vi "Media Player Example.vi"() -> ()   [LabVIEW 2017]
uses:
  Audio Player/AudioPlayer.lvclass
panel:
  in  "fileName":string[](array[string])=["beyond the horizon.mp3", "alone.mp4", "far far away.vlc", "mind me.avi"]
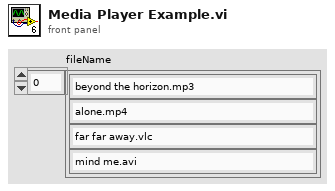
[diagram p1: front panel]
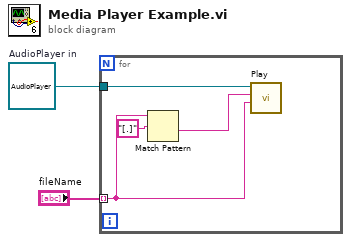
[diagram p0: block diagram]
diagram:
  w1 = refnum<class "AudioPlayer.lvclass"> refnum  # AudioPlayer in
  n1 = for {
    tunnel: "fileName" -> [w3] mode=indexing
    tunnel: w1 -> [w6]
    n2 = Match Pattern(string=w3, regular expression="[.]") -> (after substring=w4:string)  [unwired: 1 in, 3 out]
    n3 = call-dynamic "Play.vi"("fileName"=w3, "audioType"=w4, "AudioPlayer in"=w6) -> ()  [unwired: 7 in, 2 out]
  }
